vi "Init.vi"(8 "error in (no error)":errorcluster, 10 "Nb Element":u64, 11 "Slide Refnum":refnum<vi>) -> (0 "error out":errorcluster, 3 "Progress out":refnum<class "Progress.lvclass">)   [LabVIEW 2021, in "Progress.lvlib" / "Progress.lvclass"]
uses:
  Progress.lvclass
  Data.ctl
  Progress.lvclass/Progress.ctl
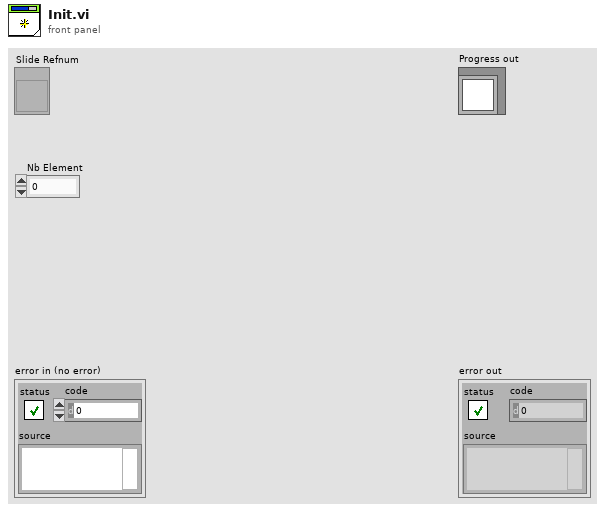
[diagram p1: front panel]
types:
  T1 = typedef "Progress.lvlib/Progress.lvclass/Data.ctl" = cluster{"SlideRefnum":refnum<vi>, "ProgressValue":u64, "NbElement":u64, "Caption":string, "UINotifier":refnum<notifier>, "StopUI":refnum<user-event>}
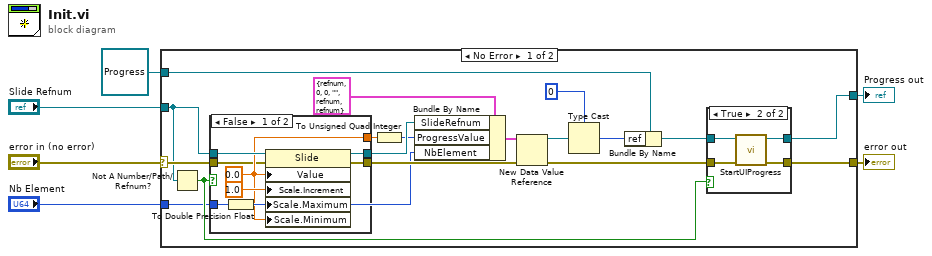
[diagram p0: block diagram]
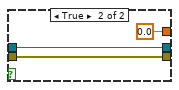
[diagram p2: hidden frame]
diagram:
  n1 = case shown="No Error" "error in (no error)" {
    selector: "error in (no error)" -> [w21 w43]
    tunnel: [w14 w43] -> w5
    tunnel: [w12 w42] -> w4
    tunnel: refnum<class "Progress.lvclass"> refnum ("Progress out") -> [w18 w42]
    tunnel: "Slide Refnum" -> [w10 _]
    tunnel: "Nb Element" -> [w7 _]
    frame No Error {
      n2 = Not A Number/Path/Refnum?(number/path/refnum=w10) -> (NaN/Path/Refnum?=w8:bool)
      n3 = case shown="False" w8 {
        tunnel: w10 -> [w32 w34]
        tunnel: w7 -> [w31 _]
        tunnel: [w29 0.0 ("ProgressValue")] -> w24
        tunnel: w21 -> [w28 w35]
        tunnel: [w27 w35] -> w20
        tunnel: [w26 w34] -> w11
        frame False {
          w29 = 0.0 ("ProgressValue")
          n4 = To Double Precision Float(number=w31) -> (double precision float=w25:dbl)
          n5 = property class="Slide"(reference=w32, error in=w28, "Value"=w29, "Scale.Increment"=1.0 ("Scale.Range:Increment"), "Scale.Maximum"=w25, "Scale.Minimum"=w29) -> (reference out=w26:refnum<vi>, error out=w27:errorcluster)
        }
        frame True {
        }
      }
      n6 = To Unsigned Quad Integer(1:w24) -> (0:w9:u64)
      n7 = Bundle By Name(cluster=T1 {"SlideRefnum"=refnum, "ProgressValue"=0, "NbElement"=0, "Caption"="", "UINotifier"=refnum, "StopUI"=refnum} ("Data"), "SlideRefnum"=w11, "ProgressValue"=w9, "NbElement"=w7) -> (w16:T1)
      n8 = New Data Value Reference(data value=w16, error in=w20) -> (data value reference=w23:refnum<data-value>, error out=w15:errorcluster)
      n9 = Type Cast(type=u64 0, x=w23) -> (*(type *) &x=w17:u64)
      n10 = Bundle By Name(cluster=w18, "ref"=w17) -> (w13:refnum<class "Progress.lvclass">)
      n11 = case shown="True" w8 {
        tunnel: w15 -> [w36 w41]
        tunnel: [w36 w40] -> w14
        tunnel: w13 -> [w37 w39]
        tunnel: [w37 w38] -> w12
        frame False {
        }
        frame True {
          n12 = call "StartUIProgress.vi"("error in (no error)"=w41, "Progress in"=w39) -> ("error out"=w40:errorcluster, "Progress out"=w38:refnum<class "Progress.lvclass">)  [unwired: 8 in]
        }
      }
    }
    frame Error {
    }
  }
  "error out" <- w5
  "Progress out" <- w4
